vi "Carriage Intake Teleop.vi"(11 "Cluster":T1) -> ()   [LabVIEW 2018]
uses:
  Support Code/Joystick Vals.ctl
  Framework/Robot Global Data.vi
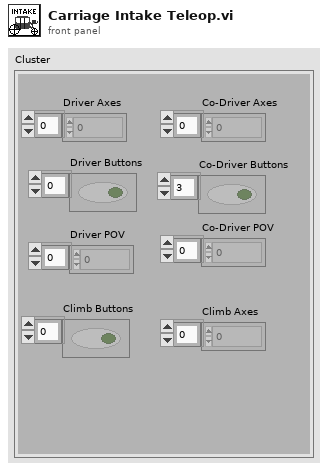
[diagram p1: front panel]
types:
  T1 = typedef "Joystick Vals.ctl" = cluster{"Driver Axes":dbl[], "Co-Driver Axes":dbl[], "Driver Buttons":bool[], "Co-Driver Buttons":bool[], "Driver POV":i16[], "Co-Driver POV":i16[], "Climb Buttons":bool[], "Climb Axes":dbl[]}
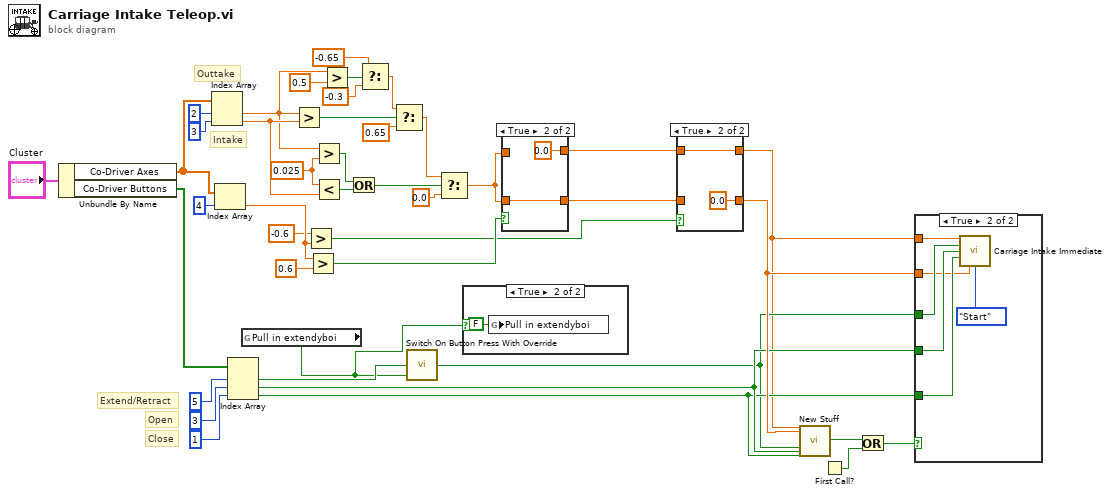
[diagram p0: block diagram]
diagram:
  w37 = 0.025 ("y")
  # "Close"
  # "Intake"
  # "Open"
  # "Extend/Retract"
  # "Outtake"
  n1 = Unbundle By Name("Cluster") -> ("Co-Driver Axes"=w16:dbl[], "Co-Driver Buttons"=w33:bool[])
  n2 = Index Array(array=w16, index #1=2 ("index"), index #2=3 ("index")) -> (element #1=w20:dbl, element #2=w24:dbl)
  n3 = Index Array(array=w16, index=4) -> (element=w13:dbl)
  n4 = Index Array(array=w33, index #1=5 ("index"), index #2=3 ("index"), index #3=1 ("index")) -> (element #1=w4:bool, element #2=w9:bool, element #3=w8:bool)
  n5 = global read "Robot Global Data.vi" "Pull in extendyboi"() -> (w2:bool)
  n6 = Greater?(x=w20, y=w24) -> (0:w23:bool)
  n7 = Greater?(x=-0.6, y=w13) -> (0:w10:bool)
  n8 = Greater?(x=w13, y=0.6) -> (0:w11:bool)
  n9 = Greater?(x=w20, y=w37) -> (0:w38:bool)
  n10 = Less?(x=w37, y=w24) -> (x < y?=w39:bool)
  n11 = Greater?(x=w20, y=0.5) -> (0:w22:bool)
  n12 = Or(x=w38, y=w39) -> (x .or. y?=w40:bool)
  n13 = Select(t=-0.65, s=w22, f=-0.3 ("t")) -> (s? t:f=w17:dbl)
  n14 = Select(t=w17, s=w23, f=0.65) -> (s? t:f=w36:dbl)
  n15 = call "Switch On Button Press With Override.vi"("Override False"=w2, "Button"=w4) -> ("Output"=w3:bool)  [unwired: 1 in]
  n16 = Select(t=w36, s=w40, f=0.0) -> (s? t:f=w32:dbl)
  n17 = case shown="True" w2 {
    frame False {
    }
    frame True {
      n18 = global write "Robot Global Data.vi" "Pull in extendyboi"(FALSE ("Pull in extendyboi")) -> ()
    }
  }
  n19 = case shown="True" w11 {
    tunnel: w32 -> [w45 _]
    tunnel: w32 -> [w44 w47]
    tunnel: [w45 0.0 ("f")] -> w31
    tunnel: [w44 w47] -> w30
    frame False {
    }
    frame True {
    }
  }
  n20 = case shown="True" w10 {
    tunnel: [w49 w51] -> w1
    tunnel: w31 -> [w49 w51]
    tunnel: [w48 0.0 ("f")] -> w29
    tunnel: w30 -> [w48 _]
    frame False {
    }
    frame True {
    }
  }
  n21 = call "New Stuff.vi"("Variant"=w1, "Variant 2"=w29, "Variant 15"=w3, "Variant 8"=w9, "Variant 7"=w8) -> ("x != y?"=w7:bool)  [unwired: 22 in]
  n22 = First Call?() -> (First Call?: T/F=w5:bool)
  n23 = Or(x=w7, y=w5) -> (x .or. y?=w6:bool)
  n24 = case shown="True" w6 {
    tunnel: w3 -> [_ w57]
    tunnel: w9 -> [_ w56]
    tunnel: w1 -> [_ w55]
    tunnel: w8 -> [_ w54]
    tunnel: w29 -> [_ w53]
    frame False {
    }
    frame True {
      n25 = call "Carriage Intake Immediate.vi"("Setpoint Left"=w55, "Extend"=w57, "Open"=w56, "Close"=w54, "Setpoint Right"=w53, "Synchronication"=enum16{"Start", "Wait"}."Start") -> ()  [unwired: 9 in, 1 out]
    }
  }
